vi "Extract Becker-Hickl ASCII Setup Parameters.vi"(8 "Error In":errorcluster, 11 "B&H Setup String":string) -> (0 "Error Out":errorcluster, 2 "Image Parameters":T2, 3 "TAC Parameters":T1 {"Frequency (Hz)" format="%#.6g"; "TAC Range (s)" format="%#.6g"; "TAC Bin (s)" format="%#.6g"})   [LabVIEW 2021, in "Becker-Hickl Files.lvlib"]
uses:
  Becker-Hickl Files.lvlib
  Becker-Hickl Setup Parameters List.ctl
  Becker-Hickl Image Parameters.ctl
  Becker-Hickl TAC Parameters.ctl
  <userlib>/_OpenG.lib/string/string.llb/openg_string.lvlib
panel:
  in  "B&H Setup Parameters":T3
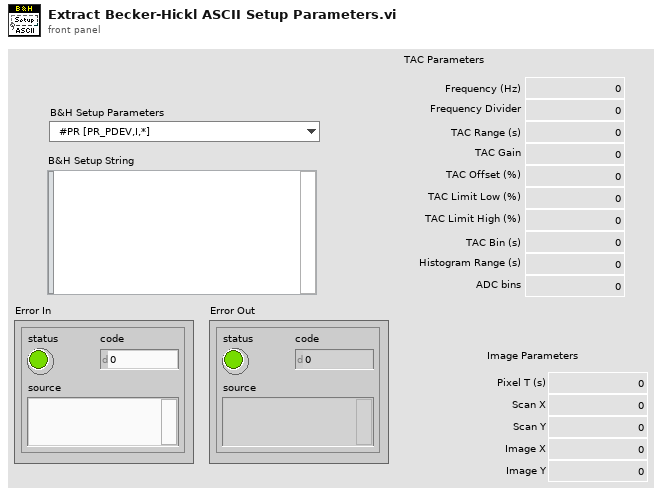
[diagram p1: front panel]
types:
  T1 = typedef "Becker-Hickl Files.lvlib/Becker-Hickl TAC Parameters.ctl" = cluster{"Frequency (Hz)":dbl, "Frequency Divider":i32, "TAC Range (s)":dbl, "TAC Gain":i32, "TAC Offset (%)":dbl, "TAC Limit Low (%)":dbl, "TAC Limit High (%)":dbl, "TAC Bin (s)":dbl, "ADC bins":i32, "Histogram Range (s)":dbl}
  T2 = typedef "Becker-Hickl Files.lvlib/Becker-Hickl Image Parameters.ctl" = cluster{"Pixel T (s)":dbl, "Scan X":i32, "Scan Y":i32, "Image X":i32, "Image Y":i32}
  T3 = typedef "Becker-Hickl Files.lvlib/Becker-Hickl Setup Parameters List.ctl" = enum16{"  #PR [PR_PDEV,I,*]", "  #PR [PR_PPORT,I,*]", "  #PR [PR_PWHAT,I,*]", "  #PR [PR_PF,B,*]", "  #PR [PR_PFNAME,S,*]", "  #PR [PR_PORIEN,I,*]", "  #PR [PR_PEJECT,B,*]", "  #PR [PR_PWIDTH,F,*]", "  #PR [PR_PHEIGH,F,*]", "  #PR [PR_PFULL,B,*]", "  #PR [PR_PAUTO,B,*]", "  #PR [PR_STP_FN,S,*]", "  #PR [PR_SAVE_T,I,*]", "  #PR [PR_SLEEP,I,*]", "  #SP [SP_MODE,I,*]", "  #SP [SP_CFD_LL,F,*]", "  #SP [SP_CFD_LH,F,*]", "  #SP [SP_CFD_ZC,F,*]", "  #SP [SP_CFD_HF,F,*]", "  #SP [SP_SYN_ZC,F,*]", "  #SP [SP_SYN_FD,I,*]", "  #SP [SP_SYN_FQ,F,*]", "  #SP [SP_SYN_HF,F,*]", "  #SP [SP_TAC_R,F,*]", "  #SP [SP_TAC_G,I,*]", "  #SP [SP_TAC_OF,F,*]", "  #SP [SP_TAC_LL,F,*]", "  #SP [SP_TAC_LH,F,*]", "  #SP [SP_TAC_TC,F,*]", "  #SP [SP_TAC_TD,F,*]", "  #SP [SP_ADC_RE,I,*]", "  #SP [SP_EAL_DE,I,*]", "  #SP [SP_NCX,I,*]", "  #SP [SP_NCY,I,*]", "  #SP [SP_PAGE,I,*]", "  #SP [SP_COL_T,F,*]", "  #SP [SP_REP_T,F,*]", "  #SP [SP_DIS_T,F,*]", "  #SP [SP_REPEAT,B,*]", "  #SP [SP_STOPT,B,*]", "  #SP [SP_OVERFL,C,*]", "  #SP [SP_WL_STA,F,*]", "  #SP [SP_WL_STO,F,*]", "  #SP [SP_WL_STE,F,*]", "  #SP [SP_EXTST,B,*]", "  #SP [SP_STEPS,I,*]", "  #SP [SP_OFFSET,F,*]", "  #SP [SP_YWIN_N,I,*]", "  #SP [SP_XWIN_N,I,*]", "  #SP [SP_TWIN_N,I,*]", "  #SP [SP_X_EQU,B,*]", "  #SP [SP_Y_EQU,B,*]", "  #SP [SP_T_EQU,B,*]", "  #SP [SP_DITH,I,*]", "  #SP [SP_EN_INT,B,*]", "  #SP [SP_INCR,I,*]", "  #SP [SP_DAES,B,*]", "  #SP [SP_SPE_FN,S,*]", "  #SP [SP_CYCLES,U,*]", "  #SP [SP_DAEC,B,*]", "  #SP [SP_MEM_BANK,I,*]", "  #SP [SP_DTCOMP,B,*]", "  #SP [SP_SCF,I,*]", "  #SP [SP_POL_L,I,*]", "  #SP [SP_POL_F,I,*]", "  #SP [SP_PIX,I,*]", "  #SP [SP_LDIV,I,*]", "  #SP [SP_ACCUM,B,*]", "  #SP [SP_ROUT,B,*]", "  #SP [SP_TAC_EH,F,*]", "  #SP [SP_DLIM,I,*]", "  #SP [SP_PHOT_F,U,*]", "  #SP [SP_EN_DLIM,B,*]", "  #SP [SP_PH_BUF,I,*]", "  #SP [SP_FLB_Y,I,*]", "  #SP [SP_FLB_X,I,*]", "  #SP [SP_BORD_U,I,*]", "  #SP [SP_BORD_L,I,*]", "  #SP [SP_POL_P,I,*]", "  #SP [SP_PIX_T,F,*]", "  #SP [SP_PIX_CLK,I,*]", "  #SP [SP_TRIGGER,I,*]", "  #SP [SP_SCAN_X,I,*]", "  #SP [SP_SCAN_Y,I,*]", "  #SP [SP_SCAN_RX,I,*]", "  #SP [SP_SCAN_RY,I,*]", "  #SP [SP_FIF_TYP,I,*]", "  #SP [SP_EPX_DIV,I,*]", "  #SP [SP_MTCLK,I,*]", "  #SP [SP_ADD_SEL,I,*]", "  #SP [SP_SXWIN_N,I,*]", "  #SP [SP_SYWIN_N,I,*]", "  #SP [SP_SX_EQU,B,*]", "  #SP [SP_SY_EQU,B,*]", "  #SP [SP_ASAVE,I,*]", "  #SP [SP_ADC_ZOOM,I,*]", "  #SP [SP_FIF_FNO,I,*]", "  #SP [SP_FCYCLES,U,*]", "  #SP [SP_XY_GAIN,I,*]", "  #SP [SP_IMG_X,I,*]", "  #SP [SP_IMG_Y,I,*]", "  #SP [SP_IMG_RX,I,*]", "  #SP [SP_IMG_RY,I,*]", "  #SP [SP_MST_CLK,I,*]", "  #SP [SP_ADC_DE,I,*]", "  #SP [SP_DET_TYP,I,*]", "  #SP [SP_X_AXIS,I,*]", "  #SP [SP_CH_EN,I,*]", "  #SP [SP_CH_SL,I,*]", "  #SP [SP_CH_F1,I,*]", "  #SP [SP_CH_F2,I,*]", "  #DI [DI_SCALE,I,*]", "  #DI [DI_MAXCNT,L,*]", "  #DI [DI_LBLINE,L,*]", "  #DI [DI_BLINE,L,*]", "  #DI [DI_GRID,B,*]", "  #DI [DI_GCOL_F,I,*]", "  #DI [DI_GCOL_B,I,*]", "  #DI [DI_TRACE,I,*]", "  #DI [DI_BOD_C,I,*]", "  #DI [DI_2DDIS,I,*]", "  #DI [DI_2DTRNO,I,*]", "  #DI [DI_3DOFFX,I,*]", "  #DI [DI_3DOFFY,I,*]", "  #DI [DI_3DINCX,I,*]", "  #DI [DI_3DCOL,I,*]", "  #DI [DI_3DMODE,I,*]", "  #DI [DI_YWIN,I,*]", "  #DI [DI_XWIN,I,*]", "  #DI [DI_TWIN,I,*]", "  #DI [DI_PSTYLE,I,*]", "  #DI [DI_PFREQ,I,*]", "  #DI [DI_CUR,B,*]", "  #DI [DI_RATE,B,*]", "  #DI [DI_2DC1,B,*]", "  #DI [DI_2DC2,B,*]", "  #DI [DI_2DC1C,I,*]", "  #DI [DI_2DC2C,I,*]", "  #DI [DI_2DC1S,I,*]", "  #DI [DI_2DC2S,I,*]", "  #DI [DI_3DC1C,I,*]", "  #DI [DI_3DC2C,I,*]", "  #DI [DI_SIZE,I,*]", "  #DI [DI_3DSTYL,I,*]", "  #DI [DI_INTCOL,I,*]", "  #DI [DI_INTPIX,I,*]", "  #DI [DI_COL_NO,I,*]", "  #DI [DI_COLMIN,I,*]", "  #DI [DI_COLMAX,I,*]", "  #DI [DI_COL2,I,*]", "  #DI [DI_COL3,I,*]", "  #DI [DI_COL4,I,*]", "  #DI [DI_COL5,I,*]", "  #DI [DI_HICOL,I,*]", "  #DI [DI_XREV,B,*]", "  #DI [DI_YREV,B,*]", "  #DI [DI_DETAIL,B,*]", "  #DI [DI_SYWIN,I,*]", "  #DI [DI_SXWIN,I,*]", "  #DI [DI_ASCALE,I,*]", "  #TR #0 [1,3342591,*]", "  #TR #1 [1,52224,*]", "  #TR #2 [1,16711680,*]", "  #TR #3 [0,13382655,*]", "  #TR #4 [0,16711935,*]", "  #TR #5 [0,3342591,*]", "  #TR #6 [0,0,*]", "  #TR #7 [0,8388608,*]", "  #WI #0 *NO *0 [0,31],*]", "  #WI #0 *NO *1 [32,63],*]", "  #WI #0 *NO *2 [64,95],*]", "  #WI #0 *NO *3 [96,127],*]", "  #WI #0 *NO *4 [128,159],*]", "  #WI #0 *NO *5 [160,191],*]", "  #WI #0 *NO *6 [192,223],*]", "  #WI #0 *NO *7 [224,255],*]", "  #WI #1 *NO *0 [0,0],*]", "  #WI #1 *NO *1 [0,0],*]", "  #WI #1 *NO *2 [0,0],*]", "  #WI #1 *NO *3 [0,0],*]", "  #WI #1 *NO *4 [0,0],*]", "  #WI #1 *NO *5 [0,0],*]", "  #WI #1 *NO *6 [0,0],*]", "  #WI #1 *NO *7 [0,0],*]", "  #WI #2 *NO *0 [0,4095],*]"}
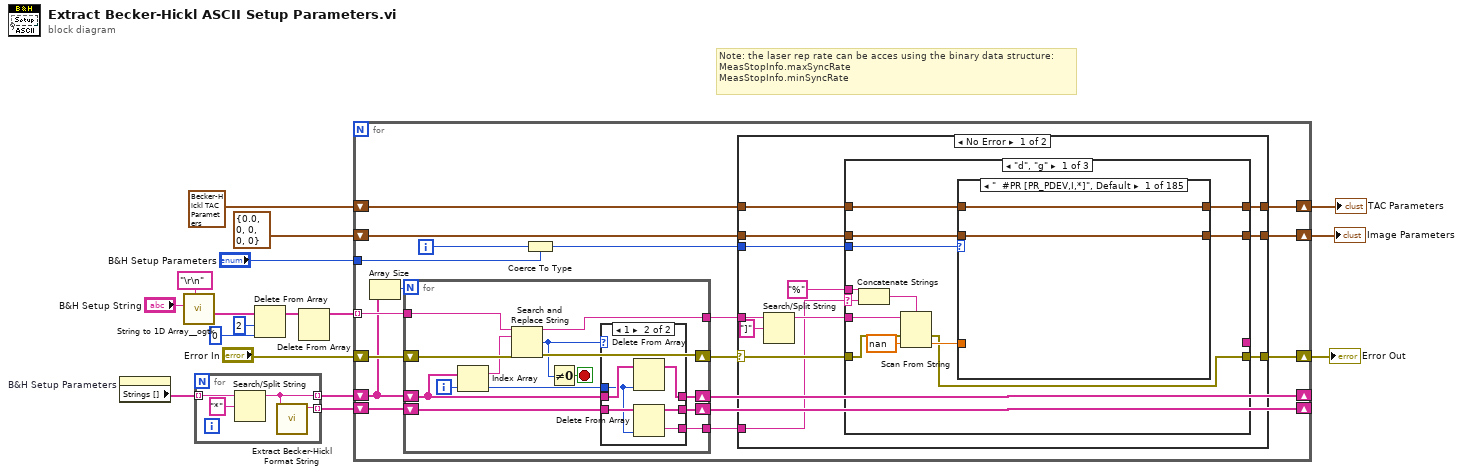
[diagram p0: block diagram]
diagram:
  # "Note: the laser rep rate can be acces using the binary data structure:\nMeasStopInfo.maxSyncRate\nMeasStopInfo.minSyncRate"
  n1 = property on="B&H Setup Parameters" class="Enum (strict)"() -> ("Strings []"=w5:string[])  [unwired: 2 in, 2 out]
  n2 = call <userlib>:"String to 1D Array__ogtk.vi"("delimiter (Tab)"="\r\n", "string"="B&H Setup String") -> ("Array of Strings"=w14:string[])  [unwired: 9 in]
  n3 = for {
    tunnel: w5 -> [w20] mode=indexing
    tunnel: [w19] -> w4 mode=indexing
    tunnel: [w18] -> w3 mode=indexing
    n4 = Search/Split String(string=w20, search string/char (-)="*") -> (substring before match=w19:string)  [unwired: 1 in, 2 out]
    n5 = call "Extract Becker-Hickl Format String.vi"("String in"=w19) -> ("Format String"=w18:string)  [unwired: 10 in]
  }
  n6 = Delete From Array(array=w14, length=2, index=0) -> (array with subset deleted=w6:string[])  [unwired: 1 out]
  n7 = Delete From Array(array=w6) -> (array with subset deleted=w7:string[])  [unwired: 2 in, 1 out]
  n8 = for {
    shift-right: [w31] -> w1
    shift-left: T1 {"Frequency (Hz)"=0.0, "Frequency Divider"=0, "TAC Range (s)"=0.0, "TAC Gain"=0, "TAC Offset (%)"=0.0, "TAC Limit Low (%)"=0.0, "TAC Limit High (%)"=0.0, "TAC Bin (s)"=0.0, "ADC bins"=0, "Histogram Range (s)"=0.0} ("TAC Parameters") -> [w32]
    shift-right: [w29] -> w9
    shift-left: "Error In" -> [w39]
    tunnel: "B&H Setup Parameters" -> [w37]
    tunnel: w7 -> [w36] mode=indexing
    shift-right: [w30] -> w10
    shift-left: T2 {"Pixel T (s)"=0.0, "Scan X"=0, "Scan Y"=0, "Image X"=0, "Image Y"=0} ("Image Parameters") -> [w33]
    shift-right: [w27] -> _
    shift-left: w4 -> [w24]
    shift-right: [w26] -> _
    shift-left: w3 -> [w28]
    i -> [w38]
    n9 = Array Size(array=w24) -> (size(s)=w23:i32)
    n10 = for {
      N: w23 -> [_]
      shift-right: [w480] -> w22
      shift-left: w39 -> [w490]
      tunnel: w36 -> [w489]
      tunnel: [w481] -> w35
      shift-right: [w485] -> w27
      shift-left: w24 -> [w487]
      shift-right: [w483] -> w26
      shift-left: w28 -> [w484]
      tunnel: [w482] -> w25
      i -> [w486]
      stop <- w478 stop-if-true
      n11 = Index Array(array=w487, index=w486) -> (element=w488:string)
      n12 = Search and Replace String(input string=w489, search string=w488, error in=w490) -> (result string=w481:string, number of replacements=w479:i32, error out=w480:errorcluster)  [unwired: 5 in, 1 out]
      n13 = Not Equal To 0?(x=w479) -> (x != 0?=w478:bool)
      n14 = case shown="1" w479 {
        tunnel: w487 -> [w492 w498]
        tunnel: w486 -> [_ w495]
        tunnel: [w492 w497] -> w485
        tunnel: w484 -> [w491 w496]
        tunnel: [w491 w494] -> w483
        tunnel: [_ w493] -> w482
        frame 0, Default {
        }
        frame 1 {
          n15 = Delete From Array(array=w498, index=w495) -> (array with subset deleted=w497:string[])  [unwired: 1 in, 1 out]
          n16 = Delete From Array(array=w496, index=w495) -> (deleted portion=w493:string, array with subset deleted=w494:string[])  [unwired: 1 in]
        }
      }
    }
    n17 = Coerce To Type(0:w38, 1:w37) -> (2:w34:T3)
    n18 = case shown="No Error" w22 {
      selector: w22 -> [w42 _]
      tunnel: w35 -> [w51 _]
      tunnel: w34 -> [w49 _]
      tunnel: w33 -> [w47 w476]
      tunnel: w32 -> [w46 w477]
      tunnel: [w45 w477] -> w31
      tunnel: [w44 w476] -> w30
      tunnel: [w43 _] -> w29
      tunnel: w25 -> [w41 _]
      frame No Error {
        n19 = Search/Split String(string=w51, search string/char (-)="]") -> (substring before match=w48:string)  [unwired: 1 in, 2 out]
        n20 = case shown="\"d\", \"g\"" w41 {
          selector: w41 -> [w54 w471 _]
          tunnel: w49 -> [w64 _ _]
          tunnel: w48 -> [w63 w472 _]
          tunnel: w47 -> [w60 w467 w474]
          tunnel: w46 -> [w59 w466 w475]
          tunnel: [w58 w466 w475] -> w45
          tunnel: [w57 w467 w474] -> w44
          tunnel: [w56 w468 w473] -> w43
          tunnel: w42 -> [w55 w469 w473]
          tunnel: [_ w465 _] -> _
          tunnel: "%" ("string") -> [w52 w463 _]
          frame "d", "g" {
            n21 = Concatenate Strings(w52, w54) -> (w53:string)
            n22 = Scan From String(format string=w53, input string=w63, error in=w55, default 1=nan ("default value 1")) -> (error out=w56:errorcluster, output 1=w61:dbl)  [unwired: 1 in, 2 out]
            n23 = case shown="\"  #PR [PR_PDEV,I,*]\", Default" w64 {
              tunnel: w61 -> [_ _ _ _ _ _ _ _ _ _ _ _ _ _ _ _ _ _ _ _ _ _ _ w113 w117 w120 w124 w130 w132 w138 w144 _ _ _ _ _ _ _ _ _ _ _ _ _ _ _ _ _ _ _ _ _ _ _ _ _ _ _ _ _ _ _ _ _ _ _ _ _ _ _ _ _ _ _ _ _ _ _ _ w243 _ _ w251 w254 _ _ _ _ _ _ _ _ _ _ _ _ _ _ _ w287 w291 _ _ _ _ _ _ _ _ _ _ _ _ _ _ _ _ _ _ _ _ _ _ _ _ _ _ _ _ _ _ _ _ _ _ _ _ _ _ _ _ _ _ _ _ _ _ _ _ _ _ _ _ _ _ _ _ _ _ _ _ _ _ _ _ _ _ _ _ _ _ _ _ _ _ _ _ _ _ _ _ _ _ _ _]
              tunnel: w60 -> [w65 w67 w69 w71 w73 w75 w77 w79 w81 w83 w85 w87 w89 w91 w93 w95 w97 w99 w101 w103 w106 w108 w109 w112 w115 w119 w123 w127 w131 w137 w141 w145 w147 w149 w151 w153 w155 w157 w159 w161 w163 w165 w167 w169 w171 w173 w175 w177 w179 w181 w183 w185 w187 w189 w191 w193 w195 w197 w199 w201 w203 w205 w207 w209 w211 w213 w215 w217 w219 w221 w223 w225 w227 w229 w231 w233 w235 w237 w239 w244 w245 w247 w252 w256 w257 w259 w261 w263 w265 w267 w269 w271 w273 w275 w277 w279 w281 w283 w285 w289 w293 w295 w297 w299 w301 w303 w305 w307 w309 w311 w313 w315 w317 w319 w321 w323 w325 w327 w329 w331 w333 w335 w337 w339 w341 w343 w345 w347 w349 w351 w353 w355 w357 w359 w361 w363 w365 w367 w369 w371 w373 w375 w377 w379 w381 w383 w385 w387 w389 w391 w393 w395 w397 w399 w401 w403 w405 w407 w409 w411 w413 w415 w417 w419 w421 w423 w425 w427 w429 w431 w433 w435 w437 w439 w441 w443 w445 w447 w449 w451 w453 w455 w457 w459 w461]
              tunnel: w59 -> [w66 w68 w70 w72 w74 w76 w78 w80 w82 w84 w86 w88 w90 w92 w94 w96 w98 w100 w102 w104 w105 w107 w110 w114 w118 w122 w126 w129 w134 w140 w143 w146 w148 w150 w152 w154 w156 w158 w160 w162 w164 w166 w168 w170 w172 w174 w176 w178 w180 w182 w184 w186 w188 w190 w192 w194 w196 w198 w200 w202 w204 w206 w208 w210 w212 w214 w216 w218 w220 w222 w224 w226 w228 w230 w232 w234 w236 w238 w240 w241 w246 w248 w249 w253 w258 w260 w262 w264 w266 w268 w270 w272 w274 w276 w278 w280 w282 w284 w286 w290 w294 w296 w298 w300 w302 w304 w306 w308 w310 w312 w314 w316 w318 w320 w322 w324 w326 w328 w330 w332 w334 w336 w338 w340 w342 w344 w346 w348 w350 w352 w354 w356 w358 w360 w362 w364 w366 w368 w370 w372 w374 w376 w378 w380 w382 w384 w386 w388 w390 w392 w394 w396 w398 w400 w402 w404 w406 w408 w410 w412 w414 w416 w418 w420 w422 w424 w426 w428 w430 w432 w434 w436 w438 w440 w442 w444 w446 w448 w450 w452 w454 w456 w458 w460 w462]
              tunnel: [w66 w68 w70 w72 w74 w76 w78 w80 w82 w84 w86 w88 w90 w92 w94 w96 w98 w100 w102 w104 w105 w107 w110 w111 w116 w121 w125 w128 w133 w139 w142 w146 w148 w150 w152 w154 w156 w158 w160 w162 w164 w166 w168 w170 w172 w174 w176 w178 w180 w182 w184 w186 w188 w190 w192 w194 w196 w198 w200 w202 w204 w206 w208 w210 w212 w214 w216 w218 w220 w222 w224 w226 w228 w230 w232 w234 w236 w238 w240 w241 w246 w248 w249 w253 w258 w260 w262 w264 w266 w268 w270 w272 w274 w276 w278 w280 w282 w284 w286 w290 w294 w296 w298 w300 w302 w304 w306 w308 w310 w312 w314 w316 w318 w320 w322 w324 w326 w328 w330 w332 w334 w336 w338 w340 w342 w344 w346 w348 w350 w352 w354 w356 w358 w360 w362 w364 w366 w368 w370 w372 w374 w376 w378 w380 w382 w384 w386 w388 w390 w392 w394 w396 w398 w400 w402 w404 w406 w408 w410 w412 w414 w416 w418 w420 w422 w424 w426 w428 w430 w432 w434 w436 w438 w440 w442 w444 w446 w448 w450 w452 w454 w456 w458 w460 w462] -> w58
              tunnel: [w65 w67 w69 w71 w73 w75 w77 w79 w81 w83 w85 w87 w89 w91 w93 w95 w97 w99 w101 w103 w106 w108 w109 w112 w115 w119 w123 w127 w131 w137 w141 w145 w147 w149 w151 w153 w155 w157 w159 w161 w163 w165 w167 w169 w171 w173 w175 w177 w179 w181 w183 w185 w187 w189 w191 w193 w195 w197 w199 w201 w203 w205 w207 w209 w211 w213 w215 w217 w219 w221 w223 w225 w227 w229 w231 w233 w235 w237 w239 w242 w245 w247 w250 w255 w257 w259 w261 w263 w265 w267 w269 w271 w273 w275 w277 w279 w281 w283 w285 w288 w292 w295 w297 w299 w301 w303 w305 w307 w309 w311 w313 w315 w317 w319 w321 w323 w325 w327 w329 w331 w333 w335 w337 w339 w341 w343 w345 w347 w349 w351 w353 w355 w357 w359 w361 w363 w365 w367 w369 w371 w373 w375 w377 w379 w381 w383 w385 w387 w389 w391 w393 w395 w397 w399 w401 w403 w405 w407 w409 w411 w413 w415 w417 w419 w421 w423 w425 w427 w429 w431 w433 w435 w437 w439 w441 w443 w445 w447 w449 w451 w453 w455 w457 w459 w461] -> w57
              frame "  #PR [PR_PDEV,I,*]", Default {
              }
              frame "  #PR [PR_PPORT,I,*]" {
              }
              frame "  #PR [PR_PWHAT,I,*]" {
              }
              frame "  #PR [PR_PF,B,*]" {
              }
              frame "  #PR [PR_PFNAME,S,*]" {
              }
              frame "  #PR [PR_PORIEN,I,*]" {
              }
              frame "  #PR [PR_PEJECT,B,*]" {
              }
              frame "  #PR [PR_PWIDTH,F,*]" {
              }
              frame "  #PR [PR_PHEIGH,F,*]" {
              }
              frame "  #PR [PR_PFULL,B,*]" {
              }
              frame "  #PR [PR_PAUTO,B,*]" {
              }
              frame "  #PR [PR_STP_FN,S,*]" {
              }
              frame "  #PR [PR_SAVE_T,I,*]" {
              }
              frame "  #PR [PR_SLEEP,I,*]" {
              }
              frame "  #SP [SP_MODE,I,*]" {
              }
              frame "  #SP [SP_CFD_LL,F,*]" {
              }
              frame "  #SP [SP_CFD_LH,F,*]" {
              }
              frame "  #SP [SP_CFD_ZC,F,*]" {
              }
              frame "  #SP [SP_CFD_HF,F,*]" {
              }
              frame "  #SP [SP_SYN_ZC,F,*]" {
              }
              frame "  #SP [SP_SYN_FD,I,*]" {
              }
              frame "  #SP [SP_SYN_FQ,F,*]" {
              }
              frame "  #SP [SP_SYN_HF,F,*]" {
              }
              frame "  #SP [SP_TAC_R,F,*]" {
                n24 = Bundle By Name(cluster=w114, "TAC Range (s)"=w113) -> (w111:T1)
              }
              frame "  #SP [SP_TAC_G,I,*]" {
                n25 = Bundle By Name(cluster=w118, "TAC Gain"=w117) -> (w116:T1)
              }
              frame "  #SP [SP_TAC_OF,F,*]" {
                n26 = Bundle By Name(cluster=w122, "TAC Offset (%)"=w120) -> (w121:T1)
              }
              frame "  #SP [SP_TAC_LL,F,*]" {
                n27 = Bundle By Name(cluster=w126, "TAC Limit Low (%)"=w124) -> (w125:T1)
              }
              frame "  #SP [SP_TAC_LH,F,*]" {
                n28 = Bundle By Name(cluster=w129, "TAC Limit High (%)"=w130) -> (w128:T1)
              }
              frame "  #SP [SP_TAC_TC,F,*]" {
                n29 = Bundle By Name(cluster=w134, "TAC Bin (s)"=w132) -> (w133:T1)
              }
              frame "  #SP [SP_TAC_TD,F,*]" {
                n30 = Compound Arithmetic op=MULTIPLY(w138, 10.0 ("value")) -> (w136:dbl)
                n31 = Bundle By Name(cluster=w140, "Histogram Range (s)"=w136) -> (w139:T1)
              }
              frame "  #SP [SP_ADC_RE,I,*]" {
                n32 = Bundle By Name(cluster=w143, "ADC bins"=w144) -> (w142:T1)
              }
              frame "  #SP [SP_EAL_DE,I,*]" {
              }
              frame "  #SP [SP_NCX,I,*]" {
              }
              frame "  #SP [SP_NCY,I,*]" {
              }
              frame "  #SP [SP_PAGE,I,*]" {
              }
              frame "  #SP [SP_COL_T,F,*]" {
              }
              frame "  #SP [SP_REP_T,F,*]" {
              }
              frame "  #SP [SP_DIS_T,F,*]" {
              }
              frame "  #SP [SP_REPEAT,B,*]" {
              }
              frame "  #SP [SP_STOPT,B,*]" {
              }
              frame "  #SP [SP_OVERFL,C,*]" {
              }
              frame "  #SP [SP_WL_STA,F,*]" {
              }
              frame "  #SP [SP_WL_STO,F,*]" {
              }
              frame "  #SP [SP_WL_STE,F,*]" {
              }
              frame "  #SP [SP_EXTST,B,*]" {
              }
              frame "  #SP [SP_STEPS,I,*]" {
              }
              frame "  #SP [SP_OFFSET,F,*]" {
              }
              frame "  #SP [SP_YWIN_N,I,*]" {
              }
              frame "  #SP [SP_XWIN_N,I,*]" {
              }
              frame "  #SP [SP_TWIN_N,I,*]" {
              }
              frame "  #SP [SP_X_EQU,B,*]" {
              }
              frame "  #SP [SP_Y_EQU,B,*]" {
              }
              frame "  #SP [SP_T_EQU,B,*]" {
              }
              frame "  #SP [SP_DITH,I,*]" {
              }
              frame "  #SP [SP_EN_INT,B,*]" {
              }
              frame "  #SP [SP_INCR,I,*]" {
              }
              frame "  #SP [SP_DAES,B,*]" {
              }
              frame "  #SP [SP_SPE_FN,S,*]" {
              }
              frame "  #SP [SP_CYCLES,U,*]" {
              }
              frame "  #SP [SP_DAEC,B,*]" {
              }
              frame "  #SP [SP_MEM_BANK,I,*]" {
              }
              frame "  #SP [SP_DTCOMP,B,*]" {
              }
              frame "  #SP [SP_SCF,I,*]" {
              }
              frame "  #SP [SP_POL_L,I,*]" {
              }
              frame "  #SP [SP_POL_F,I,*]" {
              }
              frame "  #SP [SP_PIX,I,*]" {
              }
              frame "  #SP [SP_LDIV,I,*]" {
              }
              frame "  #SP [SP_ACCUM,B,*]" {
              }
              frame "  #SP [SP_ROUT,B,*]" {
              }
              frame "  #SP [SP_TAC_EH,F,*]" {
              }
              frame "  #SP [SP_DLIM,I,*]" {
              }
              frame "  #SP [SP_PHOT_F,U,*]" {
              }
              frame "  #SP [SP_EN_DLIM,B,*]" {
              }
              frame "  #SP [SP_PH_BUF,I,*]" {
              }
              frame "  #SP [SP_FLB_Y,I,*]" {
              }
              frame "  #SP [SP_FLB_X,I,*]" {
              }
              frame "  #SP [SP_BORD_U,I,*]" {
              }
              frame "  #SP [SP_BORD_L,I,*]" {
              }
              frame "  #SP [SP_POL_P,I,*]" {
              }
              frame "  #SP [SP_PIX_T,F,*]" {
                n33 = Bundle By Name(cluster=w244, "Pixel T (s)"=w243) -> (w242:T2)
              }
              frame "  #SP [SP_PIX_CLK,I,*]" {
              }
              frame "  #SP [SP_TRIGGER,I,*]" {
              }
              frame "  #SP [SP_SCAN_X,I,*]" {
                n34 = Bundle By Name(cluster=w252, "Scan X"=w251) -> (w250:T2)
              }
              frame "  #SP [SP_SCAN_Y,I,*]" {
                n35 = Bundle By Name(cluster=w256, "Scan Y"=w254) -> (w255:T2)
              }
              frame "  #SP [SP_SCAN_RX,I,*]" {
              }
              frame "  #SP [SP_SCAN_RY,I,*]" {
              }
              frame "  #SP [SP_FIF_TYP,I,*]" {
              }
              frame "  #SP [SP_EPX_DIV,I,*]" {
              }
              frame "  #SP [SP_MTCLK,I,*]" {
              }
              frame "  #SP [SP_ADD_SEL,I,*]" {
              }
              frame "  #SP [SP_SXWIN_N,I,*]" {
              }
              frame "  #SP [SP_SYWIN_N,I,*]" {
              }
              frame "  #SP [SP_SX_EQU,B,*]" {
              }
              frame "  #SP [SP_SY_EQU,B,*]" {
              }
              frame "  #SP [SP_ASAVE,I,*]" {
              }
              frame "  #SP [SP_ADC_ZOOM,I,*]" {
              }
              frame "  #SP [SP_FIF_FNO,I,*]" {
              }
              frame "  #SP [SP_FCYCLES,U,*]" {
              }
              frame "  #SP [SP_XY_GAIN,I,*]" {
              }
              frame "  #SP [SP_IMG_X,I,*]" {
                n36 = Bundle By Name(cluster=w289, "Image X"=w287) -> (w288:T2)
              }
              frame "  #SP [SP_IMG_Y,I,*]" {
                n37 = Bundle By Name(cluster=w293, "Image Y"=w291) -> (w292:T2)
              }
              frame "  #SP [SP_IMG_RX,I,*]" {
              }
              frame "  #SP [SP_IMG_RY,I,*]" {
              }
              frame "  #SP [SP_MST_CLK,I,*]" {
              }
              frame "  #SP [SP_ADC_DE,I,*]" {
              }
              frame "  #SP [SP_DET_TYP,I,*]" {
              }
              frame "  #SP [SP_X_AXIS,I,*]" {
              }
              frame "  #SP [SP_CH_EN,I,*]" {
              }
              frame "  #SP [SP_CH_SL,I,*]" {
              }
              frame "  #SP [SP_CH_F1,I,*]" {
              }
              frame "  #SP [SP_CH_F2,I,*]" {
              }
              frame "  #DI [DI_SCALE,I,*]" {
              }
              frame "  #DI [DI_MAXCNT,L,*]" {
              }
              frame "  #DI [DI_LBLINE,L,*]" {
              }
              frame "  #DI [DI_BLINE,L,*]" {
              }
              frame "  #DI [DI_GRID,B,*]" {
              }
              frame "  #DI [DI_GCOL_F,I,*]" {
              }
              frame "  #DI [DI_GCOL_B,I,*]" {
              }
              frame "  #DI [DI_TRACE,I,*]" {
              }
              frame "  #DI [DI_BOD_C,I,*]" {
              }
              frame "  #DI [DI_2DDIS,I,*]" {
              }
              frame "  #DI [DI_2DTRNO,I,*]" {
              }
              frame "  #DI [DI_3DOFFX,I,*]" {
              }
              frame "  #DI [DI_3DOFFY,I,*]" {
              }
              frame "  #DI [DI_3DINCX,I,*]" {
              }
              frame "  #DI [DI_3DCOL,I,*]" {
              }
              frame "  #DI [DI_3DMODE,I,*]" {
              }
              frame "  #DI [DI_YWIN,I,*]" {
              }
              frame "  #DI [DI_XWIN,I,*]" {
              }
              frame "  #DI [DI_TWIN,I,*]" {
              }
              frame "  #DI [DI_PSTYLE,I,*]" {
              }
              frame "  #DI [DI_PFREQ,I,*]" {
              }
              frame "  #DI [DI_CUR,B,*]" {
              }
              frame "  #DI [DI_RATE,B,*]" {
              }
              frame "  #DI [DI_2DC1,B,*]" {
              }
              frame "  #DI [DI_2DC2,B,*]" {
              }
              frame "  #DI [DI_2DC1C,I,*]" {
              }
              frame "  #DI [DI_2DC2C,I,*]" {
              }
              frame "  #DI [DI_2DC1S,I,*]" {
              }
              frame "  #DI [DI_2DC2S,I,*]" {
              }
              frame "  #DI [DI_3DC1C,I,*]" {
              }
              frame "  #DI [DI_3DC2C,I,*]" {
              }
              frame "  #DI [DI_SIZE,I,*]" {
              }
              frame "  #DI [DI_3DSTYL,I,*]" {
              }
              frame "  #DI [DI_INTCOL,I,*]" {
              }
              frame "  #DI [DI_INTPIX,I,*]" {
              }
              frame "  #DI [DI_COL_NO,I,*]" {
              }
              frame "  #DI [DI_COLMIN,I,*]" {
              }
              frame "  #DI [DI_COLMAX,I,*]" {
              }
              frame "  #DI [DI_COL2,I,*]" {
              }
              frame "  #DI [DI_COL3,I,*]" {
              }
              frame "  #DI [DI_COL4,I,*]" {
              }
              frame "  #DI [DI_COL5,I,*]" {
              }
              frame "  #DI [DI_HICOL,I,*]" {
              }
              frame "  #DI [DI_XREV,B,*]" {
              }
              frame "  #DI [DI_YREV,B,*]" {
              }
              frame "  #DI [DI_DETAIL,B,*]" {
              }
              frame "  #DI [DI_SYWIN,I,*]" {
              }
              frame "  #DI [DI_SXWIN,I,*]" {
              }
              frame "  #DI [DI_ASCALE,I,*]" {
              }
              frame "  #TR #0 [1,3342591,*]" {
              }
              frame "  #TR #1 [1,52224,*]" {
              }
              frame "  #TR #2 [1,16711680,*]" {
              }
              frame "  #TR #3 [0,13382655,*]" {
              }
              frame "  #TR #4 [0,16711935,*]" {
              }
              frame "  #TR #5 [0,3342591,*]" {
              }
              frame "  #TR #6 [0,0,*]" {
              }
              frame "  #TR #7 [0,8388608,*]" {
              }
              frame "  #WI #0 *NO *0 [0,31],*]" {
              }
              frame "  #WI #0 *NO *1 [32,63],*]" {
              }
              frame "  #WI #0 *NO *2 [64,95],*]" {
              }
              frame "  #WI #0 *NO *3 [96,127],*]" {
              }
              frame "  #WI #0 *NO *4 [128,159],*]" {
              }
              frame "  #WI #0 *NO *5 [160,191],*]" {
              }
              frame "  #WI #0 *NO *6 [192,223],*]" {
              }
              frame "  #WI #0 *NO *7 [224,255],*]" {
              }
              frame "  #WI #1 *NO *0 [0,0],*]" {
              }
              frame "  #WI #1 *NO *1 [0,0],*]" {
              }
              frame "  #WI #1 *NO *2 [0,0],*]" {
              }
              frame "  #WI #1 *NO *3 [0,0],*]" {
              }
              frame "  #WI #1 *NO *4 [0,0],*]" {
              }
              frame "  #WI #1 *NO *5 [0,0],*]" {
              }
              frame "  #WI #1 *NO *6 [0,0],*]" {
              }
              frame "  #WI #1 *NO *7 [0,0],*]" {
              }
              frame "  #WI #2 *NO *0 [0,4095],*]" {
              }
            }
          }
          frame "s" {
            n38 = Concatenate Strings(w463, w471) -> (w464:string)
            n39 = Scan From String(format string=w464, input string=w472, error in=w469, default 1="") -> (error out=w468:errorcluster, output 1=w465:string)  [unwired: 1 in, 2 out]
          }
          frame "\u0000", Default {
          }
        }
      }
      frame Error {
      }
    }
  }
  "Error Out" <- w9
  "TAC Parameters" <- w1
  "Image Parameters" <- w10
